vi "OE 5 4 TO 16 Decoder using 3 to 8 decoder (1).vi"() -> ()   [LabVIEW 2021]
panel:
  out "Y15":bool
  out "Y14":bool
  out "Y13":bool
  out "Y12":bool
  out "Y11":bool
  out "Y10":bool
  out "Y9":bool
  out "Y8":bool
  out "Y7":bool
  out "Y6":bool
  out "Y5":bool
  out "Y4":bool
  out "Y3":bool
  out "Y2":bool
  out "Y1":bool
  out "Y0":bool
  in  "E":bool
  in  "C":bool
  in  "B":bool
  in  "A":bool
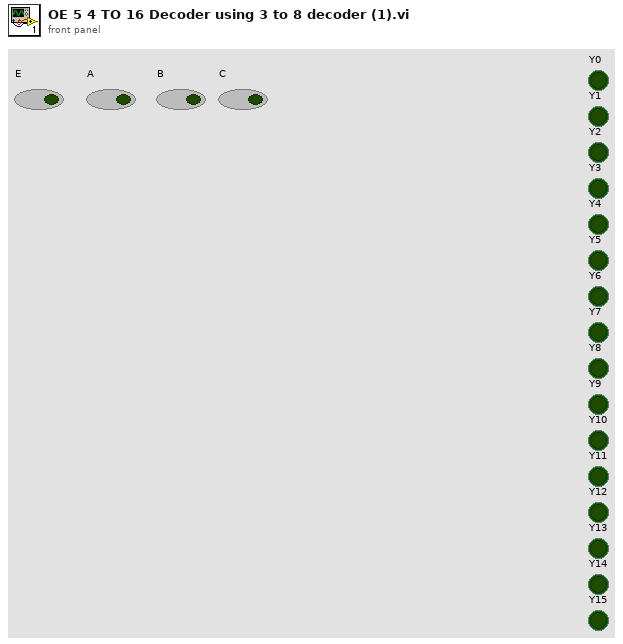
[diagram p1: front panel]
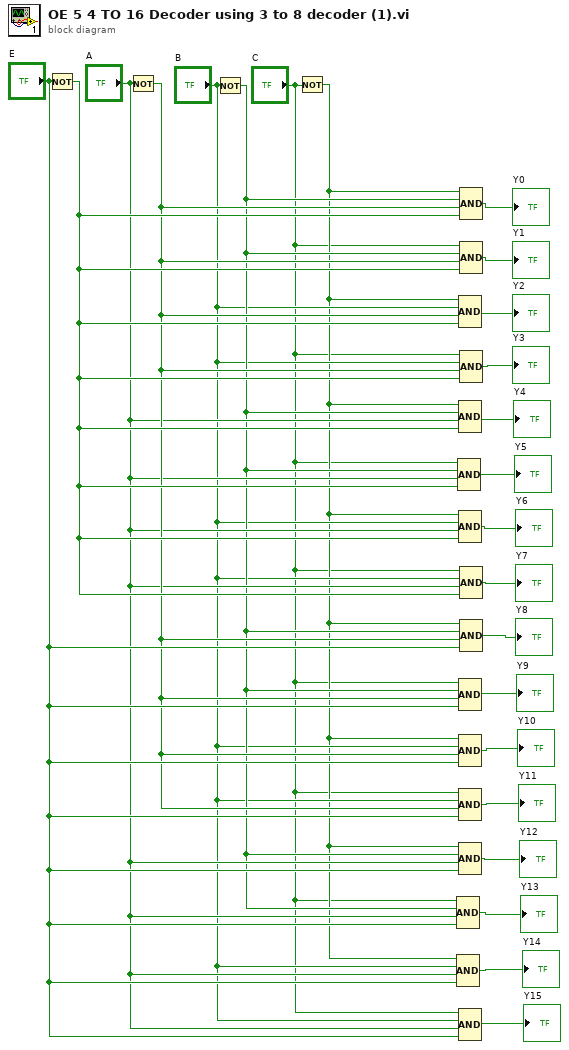
[diagram p0: block diagram]
diagram:
  n1 = Not(x="E") -> (.not. x?=w8:bool)
  n2 = Not(x="A") -> (.not. x?=w6:bool)
  n3 = Not(x="B") -> (.not. x?=w4:bool)
  n4 = Not(x="C") -> (.not. x?=w2:bool)
  n5 = Compound Arithmetic op=AND("C", w4, "A", "E") -> (→"Y13":bool)
  n6 = Compound Arithmetic op=AND(w2, "B", "A", "E") -> (→"Y14":bool)
  n7 = Compound Arithmetic op=AND("C", w4, "A", w8) -> (→"Y5":bool)
  n8 = Compound Arithmetic op=AND(w2, "B", w6, w8) -> (→"Y2":bool)
  n9 = Compound Arithmetic op=AND(w2, w4, "A", w8) -> (→"Y4":bool)
  n10 = Compound Arithmetic op=AND(w2, "B", "A", w8) -> (→"Y6":bool)
  n11 = Compound Arithmetic op=AND("C", w4, w6, "E") -> (→"Y9":bool)
  n12 = Compound Arithmetic op=AND(w2, "B", w6, "E") -> (→"Y10":bool)
  n13 = Compound Arithmetic op=AND("C", "B", w6, "E") -> (→"Y11":bool)
  n14 = Compound Arithmetic op=AND(w2, w4, "A", "E") -> (→"Y12":bool)
  n15 = Compound Arithmetic op=AND("C", "B", "A", "E") -> (→"Y15":bool)
  n16 = Compound Arithmetic op=AND(w2, w4, w6, w8) -> (→"Y0":bool)
  n17 = Compound Arithmetic op=AND("C", w4, w6, w8) -> (→"Y1":bool)
  n18 = Compound Arithmetic op=AND("C", "B", w6, w8) -> (→"Y3":bool)
  n19 = Compound Arithmetic op=AND("C", "B", "A", w8) -> (→"Y7":bool)
  n20 = Compound Arithmetic op=AND(w2, w4, w6, "E") -> (→"Y8":bool)
